vi "Close_BP4610.vi"(8 "error in":errorcluster, 11 "VISA":refnum<visa-resource-name> caption="VISAsession") -> (0 "error out":errorcluster)   [LabVIEW 2019]
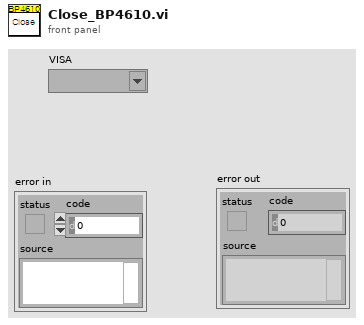
[diagram p1: front panel]
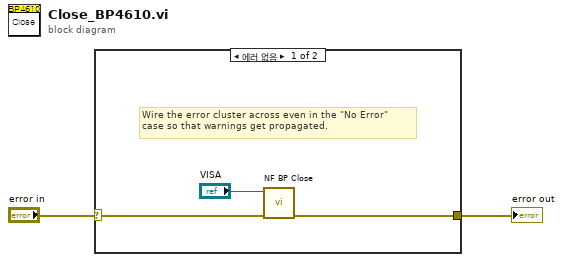
[diagram p0: block diagram]
diagram:
  n1 = case shown="에러 없음" "error in" {
    selector: "error in" -> [w5 w6]
    tunnel: [w4 w6] -> w1
    frame No Error {
      # "Wire the error cluster across even in the \"No Error\"\ncase so that warnings get propagated."
      n2 = call <instrlib>:"NF BP Close.vi"("error in (no error)"=w5, "VISAsession"="VISA") -> ("error out"=w4:errorcluster)  [unwired: 9 in]
    }
    frame Error {
    }
  }
  "error out" <- w1
